vi "RSZVB Set AUX Fixed Power.vi"(8 "error in (no error)":errorcluster {"code" format="%.0x"}, 9 "Fixed Power (-25.0)":dbl=-25.0 format="%^.3e", 10 "Channel (1)":i32=1, 11 "VISA session":refnum<visa-resource-name>) -> (0 "error out":errorcluster {"code" format="%.0x"}, 3 "dup VISA session":refnum<visa-resource-name>)   [LabVIEW 2011]
doc: "Defines a fixed power for the Aux LO signal in a vector mixer measurement (option R&S ZVA-K5). The Aux LO signal is fed to the MEAS and REF mixers.\n\nRemote-control command(s):\nSOURce<Ch>:FREQuency:CONVersion:MIXer:PAFixed"
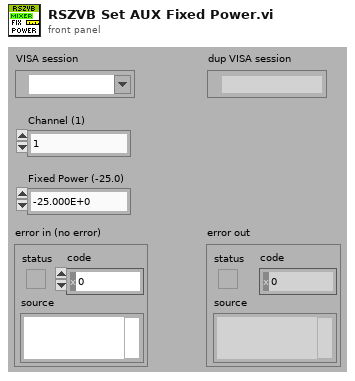
[diagram p1: front panel]
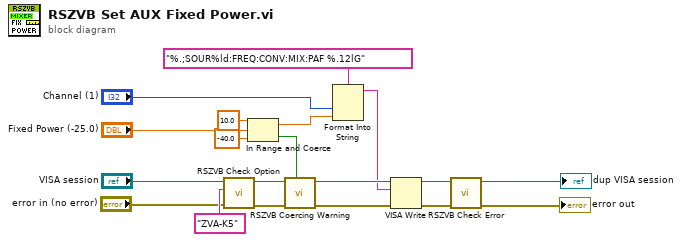
[diagram p0: block diagram]
diagram:
  n1 = call "RSZVB Check Option.vi"("error in (no error)"="error in (no error)", "Options"="ZVA-K5", "VISA session"="VISA session") -> ("error out"=w15:errorcluster, "dup VISA session"=w14:refnum<visa-resource-name>)  [unwired: 7 in]
  n2 = In Range and Coerce(upper limit=10.0, x="Fixed Power (-25.0)", lower limit=-40.0) -> (coerced(x)=w12:dbl, In Range?=w16:bool)
  n3 = call "RSZVB Coercing Warning.vi"("In Range?"=w16, "error in (no error)"=w15, "VISA session"=w14) -> ("error out"=w11:errorcluster, "dup VISA session"=w10:refnum<visa-resource-name>)  [unwired: 7 in]
  n4 = Format Into String(format string="%.;SOUR%ld:FREQ:CONV:MIX:PAF %.12lG", "Channel (1)", w12) -> (resulting string=w9:string)  [unwired: 2 in, 1 out]
  n5 = VISA Write(VISA resource name=w10, write buffer=w9, error in (no error)=w11) -> (VISA resource name out=w7:refnum<visa-resource-name>, error out=w8:errorcluster)  [unwired: 1 out]
  n6 = call "RSZVB Check Error.vi"("error in (no error)"=w8, "VISA session"=w7) -> ("error out"=→"error out":errorcluster, "dup VISA session"=→"dup VISA session":refnum<visa-resource-name>)  [unwired: 8 in]
